vi "delta_x.vi"(2 "x":dbl) -> (0 "dx":dbl)   [LabVIEW 2020]
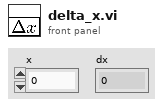
[diagram p1: front panel]
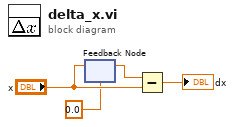
[diagram p0: block diagram]
diagram:
  n1 = feedback-in #1("x") -> ()
  n2 = feedback #1(0.0 ("Numeric")) -> (w4:dbl)
  n3 = Subtract(x=w4, y="x") -> (x-y=→"dx":dbl)
